vi "FPGA main.vi"() -> ()   [LabVIEW 2015]
uses:
  <vilib>/rvi/Emulation/niFpgaGetClockAttributes.vi
  <vilib>/rvi/Emulation/niFpgaSctlEmulationGetInTimedLoop.vi
  <vilib>/rvi/Emulation/niFpgaEmulationReportErrorSimple.vi
  <vilib>/rvi/eio/common/nirviEmuTemplateMethod_errors.vi
  <vilib>/rvi/Emulation/niFpgaCriticalErrorInLSC.vi
  <vilib>/eio/EIONode/EIONode.xnode
panel:
  in  "Valvula proporcional 2":fxp<+/-,20,5>
  in  "Valvula proporcional 1":fxp<+/-,20,5>
  in  "Temporização FPGA":u32=10000 caption="Tempo de despejo de emergência"
  in  "Tempo de despejo de emergência (mSec)":u32=10000 caption="Tempo de despejo de emergência"
  in  "Solenoide 4":bool
  in  "Solenoide 3":bool
  in  "Solenoide 2":bool
  in  "Solenoide 1":bool
  in  "Bomba 2":fxp<+/-,20,5>
  in  "Bomba 1":fxp<+/-,20,5>
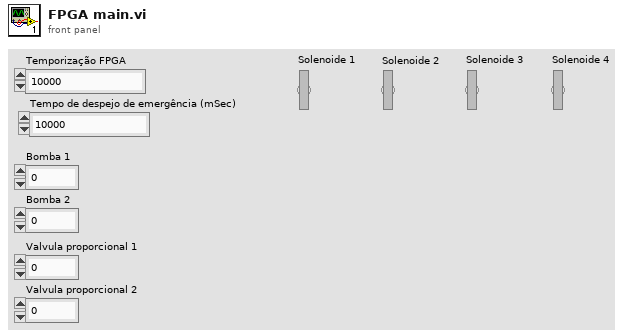
[diagram p1: front panel]
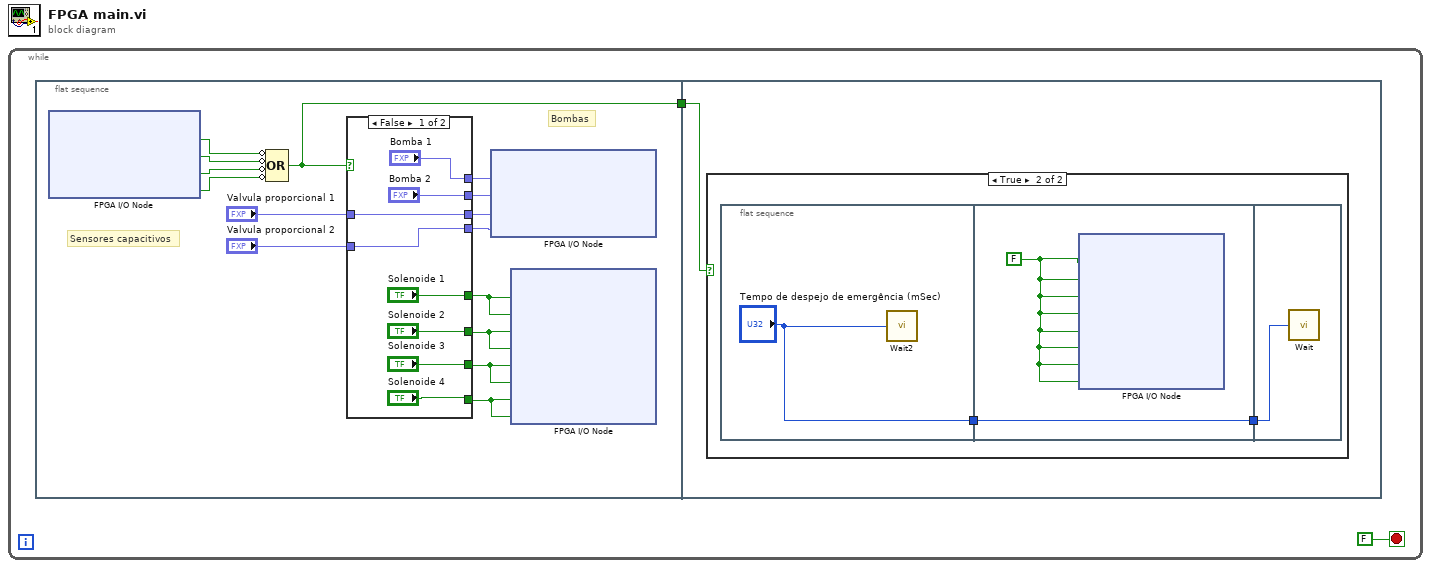
[diagram p0: block diagram]
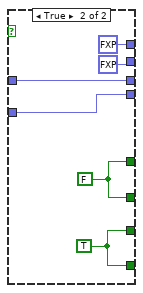
[diagram p2: hidden frame]
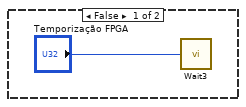
[diagram p3: hidden frame]
diagram:
  n1 = while {
    stop <- FALSE stop-if-true
    n2 = flat-sequence {
      tunnel: [w9] -> w1
      tunnel: w1 -> [w32]
      frame #0 {
        # "Bombas"
        # "Sensores capacitivos"
        n3 = xnode "FPGA I/O Node"() -> ("Entradas digitais/DI0"=w17:bool, "Entradas digitais/DI1"=w16:bool, "Entradas digitais/DI2"=w15:bool, "Entradas digitais/DI3"=w14:bool)  [unwired: 4 in, 4 out]
        n4 = Compound Arithmetic op=OR(invert w17, invert w16, invert w15, invert w14) -> (w9:bool)
        n5 = case shown="False" w9 {
          tunnel: ["Bomba 1" fxp<+/-,20,5> 0.0 ("Saídas Analógicas/AO0")] -> w13
          tunnel: ["Bomba 2" fxp<+/-,20,5> 0.0 ("Saídas Analógicas/AO1")] -> w12
          tunnel: ["Solenoide 1" w29] -> w11
          tunnel: ["Solenoide 2" w29] -> w10
          tunnel: ["Solenoide 3" w28] -> w8
          tunnel: ["Solenoide 4" w28] -> w7
          tunnel: [w19 w27] -> w5
          tunnel: "Valvula proporcional 1" -> [w19 w27]
          tunnel: [w18 w26] -> w4
          tunnel: "Valvula proporcional 2" -> [w18 w26]
          frame False {
          }
          frame True {
            w28 = TRUE ("Solenoide 1")
            w29 = FALSE ("Solenoide 1")
          }
        }
        n6 = xnode "FPGA I/O Node"("Saídas Analógicas/AO0"=w13, "Saídas Analógicas/AO1"=w12, "Saídas Analógicas/AO2"=w5, "Saídas Analógicas/AO3"=w4) -> ()  [unwired: 4 in, 4 out]
        n7 = xnode "FPGA I/O Node"("Saídas digitais/DO0"=w11, "Saídas digitais/DO1"=w11, "Saídas digitais/DO2"=w10, "Saídas digitais/DO3"=w10, "Saídas digitais/DO4"=w8, "Saídas digitais/DO5"=w8, "Saídas digitais/DO6"=w7, "Saídas digitais/DO7"=w7) -> ()  [unwired: 8 in, 8 out]
      }
      frame #1 {
        n8 = case shown="True" w32 {
          frame False {
            n9 = call "Wait3"("Count(mSec)"="Temporização FPGA") -> ()  [unwired: 1 out]
          }
          frame True {
            n10 = flat-sequence {
              tunnel: ["Tempo de despejo de emergência (mSec)"] -> w35
              tunnel: w35 -> [w38]
              tunnel: [w38] -> w34
              tunnel: w34 -> [w39]
              frame #0 {
                n11 = call "Wait2"("Count(mSec)"="Tempo de despejo de emergência (mSec)") -> ()  [unwired: 1 out]
              }
              frame #1 {
                w37 = FALSE ("Solenoide 1")
                n12 = xnode "FPGA I/O Node"("Saídas digitais/DO0"=w37, "Saídas digitais/DO1"=w37, "Saídas digitais/DO2"=w37, "Saídas digitais/DO3"=w37, "Saídas digitais/DO4"=w37, "Saídas digitais/DO5"=w37, "Saídas digitais/DO6"=w37, "Saídas digitais/DO7"=w37) -> ()  [unwired: 8 in, 8 out]
              }
              frame #2 {
                n13 = call "Wait"("Count(mSec)"=w39) -> ()  [unwired: 1 out]
              }
            }
          }
        }
      }
    }
  }
